vi "RS232_Port_ID.vi"() -> ()   [LabVIEW 2013]
doc: "This example performs writes and reads on a serial port, as directed by the user. You can press the Write and Read buttons, and change the Read Count, while the example is running.\n\nThe parameters set for the serial port must match the parameters of the connected instrument or device. In this example, the Read Count parameter specifies the number of bytes that the serial port reads. If there were more bytes at the port than the specified number, those bytes would not be read. If there were less bytes at the port than the specified number, you would receive a timeout error.\n\nThis example expands upon the flow control options for XON and XOFF, allowing the user to choose those control characters. Also, the user can enable or disable a termination character. Some devices require a termination character in order to identify the end of command strings. Some devices send a termination character to signify the end of data to be read. This example shows how you can end the Read operation once a termination character is detected in the buffer and/or append a termination character at the end of the Write data."
uses:
  <vilib>/Instr/_visa.llb/VISA Configure Serial Port (Instr).vi
  <vilib>/regexp/Match Regular Expression.xnode
panel:
  in  "Tab Control":enum32{"Page 1", "com settings"}(tab)
  out "find list":string[](array[string])=["ASRL1::INSTR", "ASRL3::INSTR", "ASRL4::INSTR", "ASRL5::INSTR", "ASRL6::INSTR"]
  in  "Stop":bool
  in  "Serial Settings":T1={"baud rate"=9600, "data bits"=7, "parity"=enum."Odd", "stop bits"=10, "flow control"=0} {"flow control" items=["None"=0, "XON/XOFF"=1, "RTS/CTS"=2, "DTR/DSR"=4]; "stop bits" items=["1.0"=10, "1.5"=15, "2.0"=20]; "data bits" min=5 max=8 step=1; "baud rate" items=["75"=75, "110"=110, "134"=134, "150"=150, "300"=300, "600"=600, "1200"=1200, "1800"=1800, "2400"=2400, "4800"=4800, "7200"=7200, "9600"=9600, "14400"=14400, "19200"=19200, "28800"=28800, "38400"=38400, "56000"=56000, "57600"=57600, "115200"=115200, "128000"=128000, "230400"=230400]}
  in  "End Read on Termination Character?":bool=TRUE
  in  "End Write on Termination Character?":bool=TRUE
  in  "XON/XOFF Characters":T2={"XON"=enum."DC1", "XOFF"=enum."DC3"}
  in  "Termination Character":u8=13 format="%.0x"
  in  "Command":string="\\n\n\\n\n\\n\n\\n\n\\n"
  # "0xA is equivalent to a '\\n' character, which is a line feed."
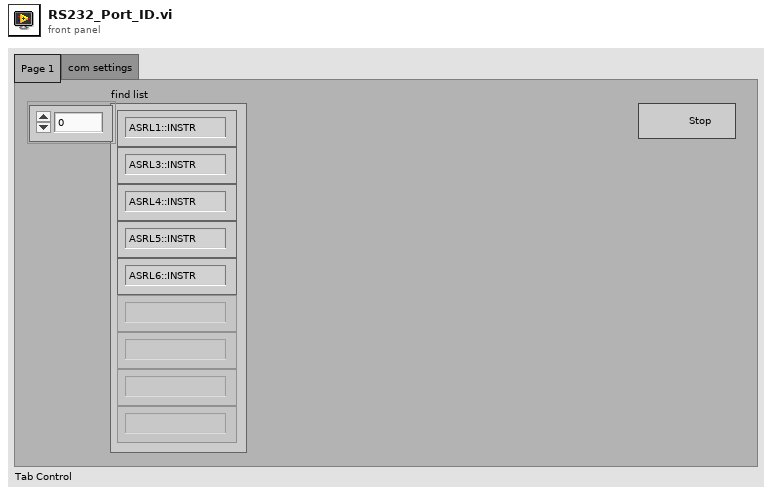
[diagram p1: front panel]
types:
  T1 = cluster{"baud rate":u32, "data bits":u16, "parity":enum16{"None", "Odd", "Even", "Mark", "Space"}, "stop bits":u16, "flow control":u16}
  T2 = cluster{"XON":enum16{"NUL", "SOH", "STX", "ETX", "EOT", "ENQ", "ACK", "BEL", "BS", "HT", "LF", "VT", "FF", "CR", "SO", "SI", "DLE", "DC1", "DC2", "DC3", "DC4", "NAK", "SYN", "ETB", "CAN", "EM", "SUB", "ESC", "FS", "GS", "RS", "US", "SP", "!", "\"", "#", "$", "%", "&", "'", "(", ")", "*", "+", ",", "- (-)", ".", "/", "0", "1", "2", "3", "4", "5", "6", "7", "8", "9", ":", ";", "<", "=", ">", "?", "@", "A", "B", "C", "D", "E", "F", "G", "H", "I", "J", "K", "L", "M", "N", "O", "P", "Q", "R", "S", "T", "U", "V", "W", "X", "Y", "Z", "[", "\\", "]", "^", "_", "`", "a", "b", "c", "d", "e", "f", "g", "h", "i", "j", "k", "l", "m", "n", "o", "p", "q", "r", "s", "t", "u", "v", "w", "x", "y", "z", "{", "|", "}", "~"}, "XOFF":enum16{"NUL", "SOH", "STX", "ETX", "EOT", "ENQ", "ACK", "BEL", "BS", "HT", "LF", "VT", "FF", "CR", "SO", "SI", "DLE", "DC1", "DC2", "DC3", "DC4", "NAK", "SYN", "ETB", "CAN", "EM", "SUB", "ESC", "FS", "GS", "RS", "US", "SP", "!", "\"", "#", "$", "%", "&", "'", "(", ")", "*", "+", ",", "- (-)", ".", "/", "0", "1", "2", "3", "4", "5", "6", "7", "8", "9", ":", ";", "<", "=", ">", "?", "@", "A", "B", "C", "D", "E", "F", "G", "H", "I", "J", "K", "L", "M", "N", "O", "P", "Q", "R", "S", "T", "U", "V", "W", "X", "Y", "Z", "[", "\\", "]", "^", "_", "`", "a", "b", "c", "d", "e", "f", "g", "h", "i", "j", "k", "l", "m", "n", "o", "p", "q", "r", "s", "t", "u", "v", "w", "x", "y", "z", "{", "|", "}", "~"}}
  T3 = enum16{"NUL", "SOH", "STX", "ETX", "EOT", "ENQ", "ACK", "BEL", "BS", "HT", "LF", "VT", "FF", "CR", "SO", "SI", "DLE", "DC1", "DC2", "DC3", "DC4", "NAK", "SYN", "ETB", "CAN", "EM", "SUB", "ESC", "FS", "GS", "RS", "US", "SP", "!", "\"", "#", "$", "%", "&", "'", "(", ")", "*", "+", ",", "- (-)", ".", "/", "0", "1", "2", "3", "4", "5", "6", "7", "8", "9", ":", ";", "<", "=", ">", "?", "@", "A", "B", "C", "D", "E", "F", "G", "H", "I", "J", "K", "L", "M", "N", "O", "P", "Q", "R", "S", "T", "U", "V", "W", "X", "Y", "Z", "[", "\\", "]", "^", "_", "`", "a", "b", "c", "d", "e", "f", "g", "h", "i", "j", "k", "l", "m", "n", "o", "p", "q", "r", "s", "t", "u", "v", "w", "x", "y", "z", "{", "|", "}", "~"}
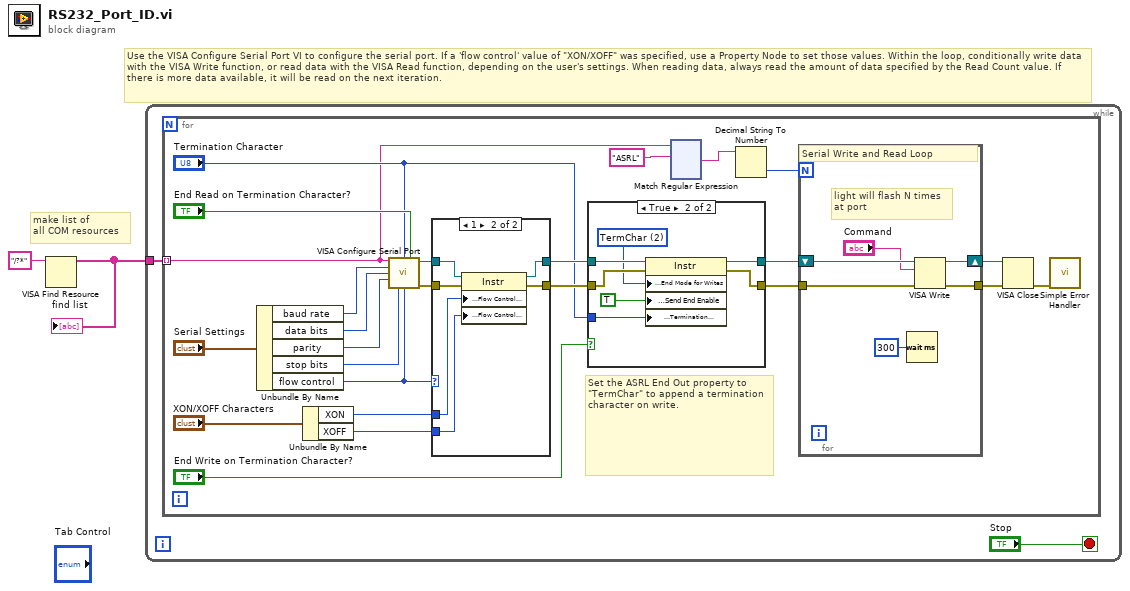
[diagram p0: block diagram]
diagram:
  # "make list of\nall COM resources"
  # "Use the VISA Configure Serial Port VI to configure the serial port. If a 'flow control' value of \"XON/XOFF\" was specified, use a Property Node to set those values. Within the loop, conditionally write data with the VISA Write function, or read data with the VISA Read function, depending on the user's settings. When reading data, always read the amount of data specified by the Read Count value. If there is more data available, it will be read on the next iteration."
  n1 = VISA Find Resource(11:"/?*" ("expression (\"?*\")")) -> (3:w1:string[])  [unwired: 2 in, 2 out]
  "find list" <- w1
  n2 = while {
    tunnel: w1 -> [w4]
    stop <- "Stop" stop-if-true
    n3 = for {
      tunnel: w4 -> [w8] mode=indexing
      # "Set the ASRL End Out property to \"TermChar\" to append a termination character on write."
      n4 = Unbundle By Name("Serial Settings") -> ("baud rate"=w23:u32, "data bits"=w24:u16, "parity"=w25:enum16{"None", "Odd", "Even", "Mark", "Space"}, "stop bits"=w26:u16, "flow control"=w17:u16)
      n5 = Unbundle By Name("XON/XOFF Characters") -> ("XON"=w16:T3, "XOFF"=w15:T3)
      n6 = call-poly "VISA Configure Serial Port"("VISA resource name"=w8, "termination char\n(0xA = '\\n' = LF)"="Termination Character", "Enable Termination\nChar (T)"="End Read on Termination Character?", "baud rate (9600)"=w23, "data bits (8)"=w24, "parity (0:none)"=w25, "stop bits (10: 1 bit)"=w26, "flow control (0:none)"=w17) -> ("VISA resource name out"=w27:refnum<visa-resource-name>, "error out"=w28:errorcluster)  [unwired: 2 in, 4 out]
      n7 = case shown="1" w17 {
        tunnel: [w159 w166] -> w14
        tunnel: [w160 w165] -> w12
        tunnel: w28 -> [w159 w164]
        tunnel: w27 -> [w160 w163]
        tunnel: w16 -> [_ w162]
        tunnel: w15 -> [_ w161]
        frame Default {
        }
        frame 1 {
          n8 = property class="Instr"(reference=w163, error in=w164, "Serial Settings:Flow Control XON Character"=w162, "Serial Settings:Flow Control XOFF Character"=w161) -> (reference out=w165:refnum<visa-resource-name>, error out=w166:errorcluster)
        }
      }
      n9 = case shown="True" "End Write on Termination Character?" {
        tunnel: w12 -> [w150 w158]
        tunnel: w14 -> [w151 w157]
        tunnel: [w150 w156] -> w11
        tunnel: [w151 w155] -> w13
        tunnel: "Termination Character" -> [_ w153]
        frame False {
        }
        frame True {
          w154 = u16 2 items=["None", "LastBit", "TermChar", "Break"] ("Serial Settings:Serial End Mode for Writes")
          n10 = property class="Instr"(reference=w158, error in=w157, "Serial Settings:End Mode for Writes"=w154, "Message Based Settings:Send End Enable"=TRUE, "Message Based Settings:Termination Character"=w153) -> (reference out=w156:refnum<visa-resource-name>, error out=w155:errorcluster)
        }
      }
      n11 = xnode "Match Regular Expression"("input string"=w8, "regular expression"="ASRL") -> ("after match"=w5:string)  [unwired: 4 in, 4 out]
      n12 = Decimal String To Number(string=w5) -> (number=w6:i32)  [unwired: 2 in, 1 out]
      n13 = for {
        N: w6 -> [_]
        shift-right: [w147] -> w18
        shift-left: w11 -> [w149]
        tunnel: w13 -> [w148]
        tunnel: [w146] -> w19
        # "light will flash N times\nat port"
        # "Serial Write and Read Loop"
        n14 = Wait (ms)(milliseconds to wait=u32 300) -> ()  [unwired: 1 out]
        n15 = VISA Write(VISA resource name=w149, write buffer="Command", error in (no error)=w148) -> (VISA resource name out=w147:refnum<visa-resource-name>, error out=w146:errorcluster)  [unwired: 1 out]
      }
      n16 = VISA Close(VISA resource name=w18, error in (no error)=w19) -> (error out=w20:errorcluster)
      n17 = call <vilib>:"Simple Error Handler.vi"("error in (no error)"=w20) -> ()  [unwired: 1 in, 8 out]
    }
  }
